vi "CalculateAveragedFFT.vi"(6 "QueuedDataInput":T6, 7 "Logging Settings Input":T4) -> (2 "FFT Cluster Output":T3[](array[typedef]), 3 "Logging Settings Output":T4)   [LabVIEW 2022 SP3]
uses:
  Logging/Logging Configuration.ctl
  TDMS-Refs.ctl
  Logging/QueuedLoggedData.ctl
  FFT-Data.ctl
  <vilib>/Analysis/4window.llb/windowTd.ctl
  <vilib>/Waveform/WDTOps.llb/WDT Get Waveform Time Array DBL.vi
  Logging/Logging.lvlib
  <vilib>/Analysis/NI_AALPro.lvlib
panel:
  in  "averaging parameters":T1={"averaging mode"=enum."Vector averaging", "weighting mode"=enum."Linear", "number of averages"=2}
  in  "window":T2=1 items=["Rectangle"=0, "Hanning"=1, "Hamming"=2, "Blackman-Harris"=3, "Exact Blackman"=4, "Blackman"=5, "Flat Top"=6, "4 Term B-Harris "=7, "7 Term B-Harris"=8, "Low Sidelobe"=9, "Blackman Nuttall"=11, "Triangle"=30, "Bartlett-Hanning"=31, "Bohman"=32, "Parzen"=33, "Welch"=34, "Kaiser"=60, "Dolph-Chebyshev"=61, "Gaussian"=62]
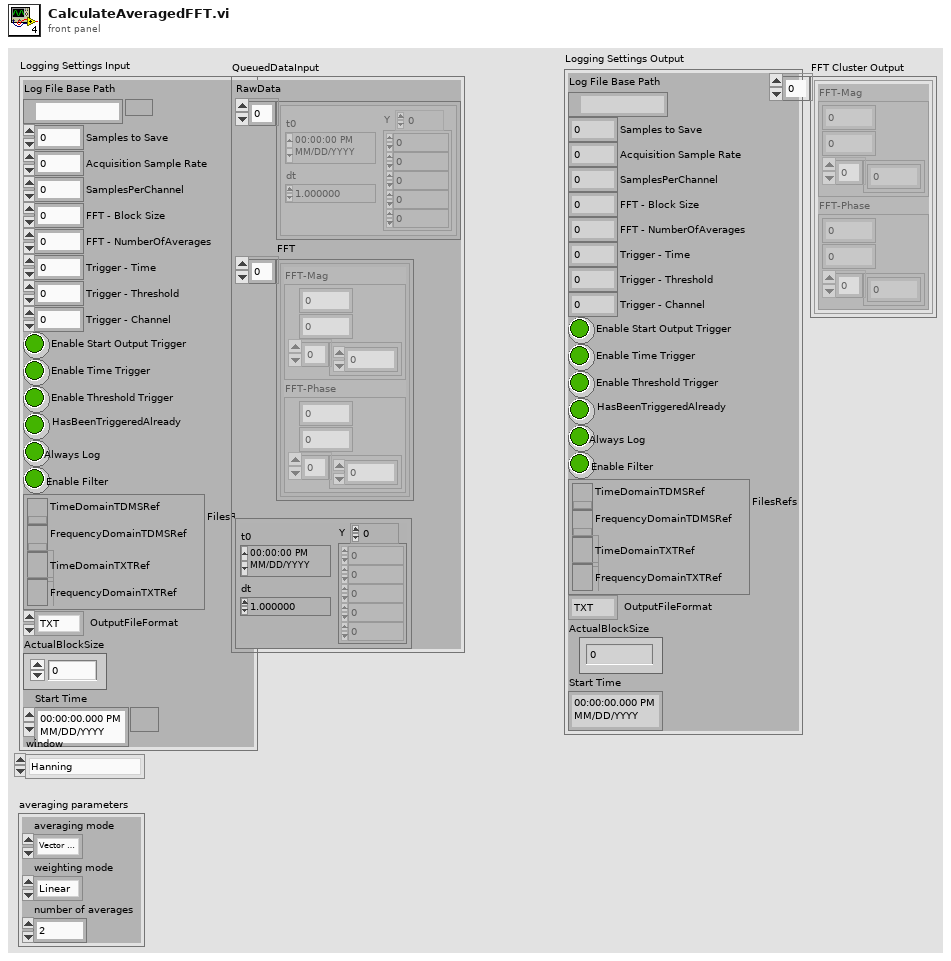
[diagram p1: front panel]
types:
  T1 = cluster{"averaging mode":enum16{"No averaging", "Vector averaging", "RMS averaging", "Peak hold"}, "weighting mode":enum16{"Linear", "Exponential"}, "number of averages":u32}
  T2 = typedef "NI_AALPro.lvlib/windowTd.ctl" = u32
  T3 = typedef "FFT-Data.ctl" = cluster{"FFT-Mag":cluster{"t0":dbl, "dt":dbl, "Y":dbl[]}, "FFT-Phase":cluster{"t0":dbl, "dt":dbl, "Y":dbl[]}}
  T4 = typedef "Logging.lvlib/Logging Configuration.ctl" = cluster{"Log File Base Path":path, "Samples to Save":u32, "Acquisition Sample Rate":dbl, "SamplesPerChannel":u32, "FFT - Block Size":u32, "FFT - NumberOfAverages":i32, "Trigger - Time":i32, "Trigger - Threshold":dbl, "Trigger - Channel":i32, "Enable Start Output Trigger":bool, "Enable Time Trigger":bool, "Enable Threshold Trigger":bool, "HasBeenTriggeredAlready":bool, "Always Log":bool, "Enable Filter":bool, "FilesRefs":T5, "OutputFileFormat":enum16{"TXT", "TDMS"}, "ActualBlockSize":i32, "Start Time":timestamp}
  T5 = typedef "TDMS-Refs.ctl" = cluster{"TimeDomainTDMSRef":refnum<k34>, "FrequencyDomainTDMSRef":refnum<k34>, "TimeDomainTXTRef":refnum<file>, "FrequencyDomainTXTRef ":refnum<file>}
  T6 = typedef "QueuedLoggedData.ctl" = cluster{"RawData":waveform(dbl)[], "FFT ":T3[], "Output Data":waveform(dbl)}
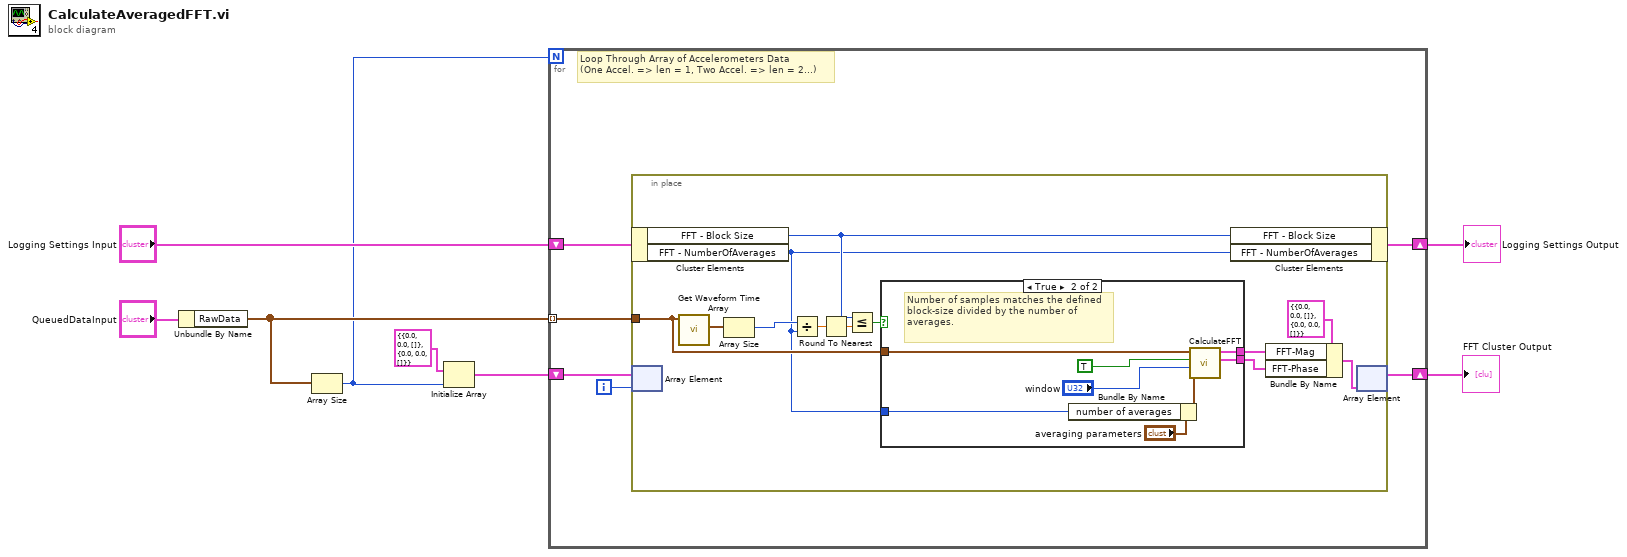
[diagram p0: block diagram]
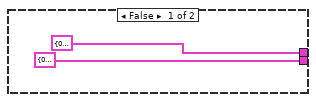
[diagram p2: hidden frame]
diagram:
  n1 = Unbundle By Name("QueuedDataInput") -> ("RawData"=w5:waveform(dbl)[])
  n2 = Array Size(array=w5) -> (size(s)=w3:i32)
  n3 = Initialize Array(T3 {"FFT-Mag"={"t0"=0.0, "dt"=0.0, "Y"=[]}, "FFT-Phase"={"t0"=0.0, "dt"=0.0, "Y"=[]}} ("FFT Cluster Input"), w3) -> (w2:T3[])
  n4 = for {
    N: w3 -> [_]
    tunnel: w5 -> [w11] mode=indexing
    shift-right: [w9] -> w6
    shift-left: "Logging Settings Input" -> [w10]
    shift-right: [w12] -> w1
    shift-left: w2 -> [w14]
    i -> [w13]
    # "Loop Through Array of Accelerometers Data\n(One Accel. => len = 1, Two Accel. => len = 2...)"
    n5 = in-place {
      in-place-border: w11 -> [w17]
      n6 = in-place-cluster #1(w10) -> ("FFT - Block Size"=w16:u32, "FFT - NumberOfAverages"=w15:i32)
      n7 = in-place-array #2(w14, w13) -> ()  [unwired: 1 out]
      n8 = call-poly <vilib>:"Get Waveform Time Array.vi"("waveform in"=w17) -> ("X array"=w26:timestamp[])  [unwired: 9 in, 1 out]
      n9 = Array Size(array=w26) -> (size(s)=w23:i32)
      n10 = Divide(x=w23, y=w15) -> (x/y=w24:dbl)
      n11 = Round To Nearest(number=w24) -> (nearest integer value=w22:dbl)
      n12 = Less Or Equal?(x=w16, y=w22) -> (x <= y?=w25:bool)
      n13 = case shown="True" w25 {
        tunnel: [cluster{dbl, dbl, dbl[]} {0.0, 0.0, []} ("FFT- Phase") w36] -> w19
        tunnel: [cluster{dbl, dbl, dbl[]} {0.0, 0.0, []} ("FFT- Mag") w35] -> w20
        tunnel: w17 -> [_ w34]
        tunnel: w15 -> [_ w29]
        frame False {
        }
        frame True {
          # "Number of samples matches the defined block-size divided by the number of averages."
          n14 = Bundle By Name(cluster="averaging parameters", "number of averages"=w29) -> (w30:T1)
          n15 = call "CalculateFFT.vi"("averaging parameters"=w30, "window"="window", "restart averaging (F)"=TRUE, "waveform"=w34) -> ("FFT- Phase"=w36:cluster{dbl, dbl, dbl[]}, "FFT- Mag"=w35:cluster{dbl, dbl, dbl[]})  [unwired: 6 in]
        }
      }
      n16 = in-place-cluster #1("FFT - Block Size"=w16, "FFT - NumberOfAverages"=w15) -> (w9:T4)
      n17 = Bundle By Name(cluster=T3 {"FFT-Mag"={"t0"=0.0, "dt"=0.0, "Y"=[]}, "FFT-Phase"={"t0"=0.0, "dt"=0.0, "Y"=[]}} ("FFTCluster"), "FFT-Mag"=w20, "FFT-Phase"=w19) -> (w18:T3)
      n18 = in-place-array #2(w18) -> (w12:T3[])  [unwired: 1 out]
    }
  }
  "Logging Settings Output" <- w6
  "FFT Cluster Output" <- w1
